vi "Write Callbacks Queue.vi"(8 "error in (no error)":errorcluster, 10 "callbacks":refnum<queue>, 11 "Future in":refnum<class "Future.lvclass">) -> (0 "error out":errorcluster, 3 "Future out":refnum<class "Future.lvclass">)   [LabVIEW 2017, in "Promise Future.lvlib" / "Future.lvclass"]
uses:
  Future.lvclass
  Future.lvclass/Future.ctl
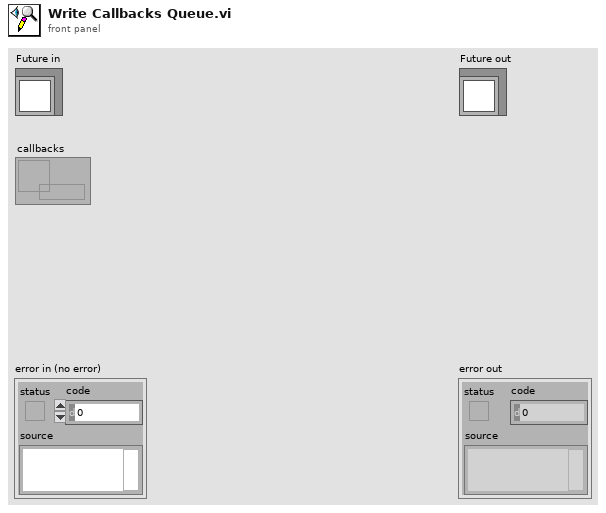
[diagram p1: front panel]
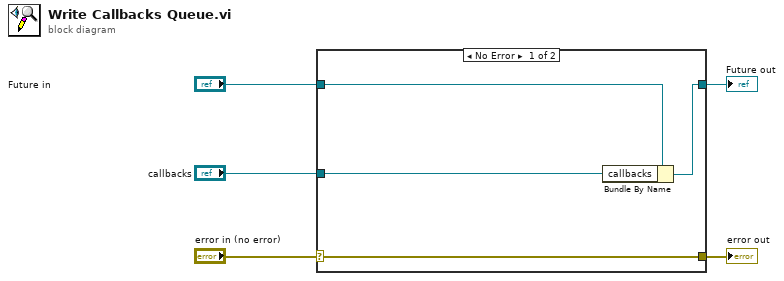
[diagram p0: block diagram]
diagram:
  n1 = case shown="No Error" "error in (no error)" {
    selector: "error in (no error)" -> [w9 w10]
    tunnel: [w9 w10] -> w4
    tunnel: [w7 w11] -> w2
    tunnel: "Future in" -> [w8 w11]
    tunnel: "callbacks" -> [w6 _]
    frame No Error {
      n2 = Bundle By Name(cluster=w8, "callbacks"=w6) -> (w7:refnum<class "Future.lvclass">)
    }
    frame Error {
    }
  }
  "error out" <- w4
  "Future out" <- w2
